vi "ui_DataLog Query Large String.vi"(0 "prompt":string, 7 "string in (\"\")":string) -> (4 "OKed?":bool, 8 "string out":string)   [LabVIEW 2012]
doc: "This dialog queries for a large string. The titlebar indicates what kind of string is expected."
uses:
  typedefs/t_DataLog Query Large String States.ctl
panel:
  in  "string":string
  in  "cancel":bool
  in  "OK":bool
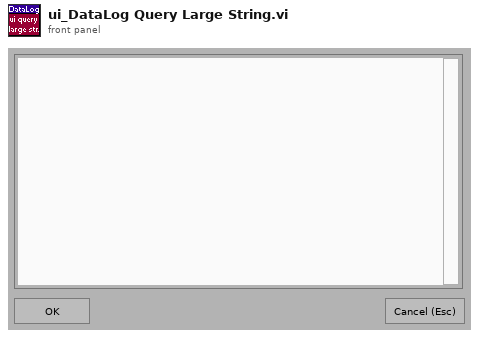
[diagram p1: front panel]
types:
  T1 = typedef "t_DataLog Query Large String States.ctl" = enum16{"empty queue", "initialize", "stop"}
  T2 = typedef "eventvkey.ctl" = enum16{"ASCII", "Enter", "Return", "Shift", "Ctrl", "Alt", "Cmd", "Opt", "Caps", "NumLock", "Clear", "Break", "Up", "Down", "Left", "Right", "Insert", "Delete", "Home", "End", "PageUp", "PageDown", "Escape", "Help", "Pause", "ScrollLock", "F1", "F2", "F3", "F4", "F5", "F6", "F7", "F8", "F9", "F10", "F11", "F12", "F13", "F14", "F15", "F16", "F17", "F18", "F19", "F20", "F21", "F22", "F23", "F24", "Play", "VolumeUp", "VolumeDown", "Mute", "Two Byte Char"}
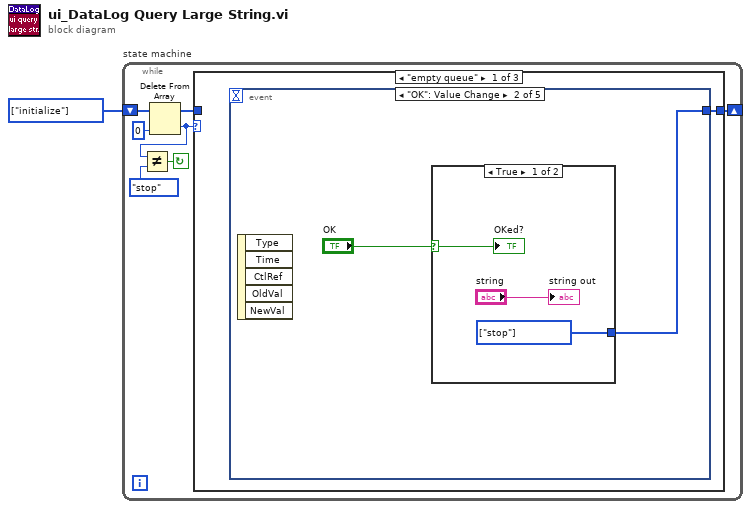
[diagram p0: block diagram]
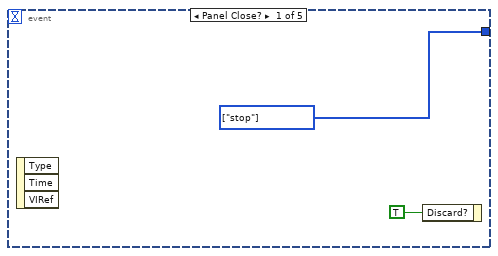
[diagram p2: hidden frame]
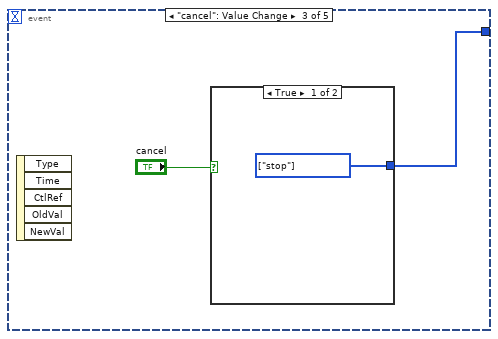
[diagram p4: hidden frame]
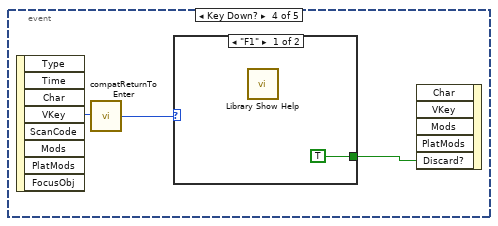
[diagram p6: hidden frame]
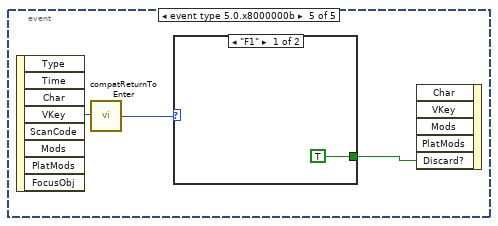
[diagram p8: hidden frame]
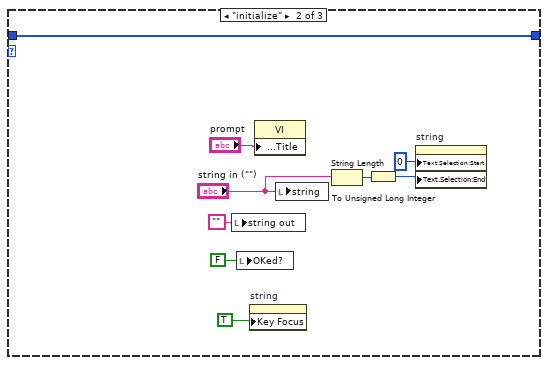
[diagram p10: hidden frame]
diagram:
  w1 = T1[] [enum."initialize"] items=["empty queue", "initialize", "stop"] ("Array Constant")
  n1 = while "state machine" {
    shift-left: w1 -> [w5]
    shift-right: [w8] -> _
    stop <- w7 continue-if-true
    n2 = Delete From Array(array=w5, index=0) -> (deleted portion=w3:T1, array with subset deleted=w4:T1[])  [unwired: 1 in]
    n3 = Not Equal?(x=w3, y=t_DataLog_Query_Large_String_States."stop" ("states")) -> (x != y?=w7:bool)
    n4 = case "Case" shown="\"empty queue\"" w3 {
      tunnel: [w9 w36 w37] -> w8
      tunnel: w4 -> [_ w36 w37]
      frame "empty queue" {
        n5 = event shown="[1] \"OK\": Value Change" {
          selector: _ -> [_ _ _ _ _]
          dyn-events: _ -> [_ _ _ _ _]
          timeout: _ -> [_ _ _ _ _]
          tunnel: [w11 w13 w18 _ _] -> w9
          event Panel Close? {
            w11 = T1[] [enum."stop"] items=["empty queue", "initialize", "stop"] ("Array Constant")
            n6 = event-data() -> ()  [unwired: 1 in, 3 out]
            n7 = event-data("Discard?"=TRUE) -> ()  [unwired: 1 in, 1 out]
          }
          event "OK": Value Change {
            n8 = event-data() -> ()  [unwired: 1 in, 5 out]
            n9 = case shown="True" "OK" {
              selector: "OK" -> [w14 _]
              tunnel: [w16 _] -> w13
              frame True {
                w16 = T1[] [enum."stop"] items=["empty queue", "initialize", "stop"] ("Array Constant")
                "string out" <- "string"
                "OKed?" <- w14
              }
              frame False {
              }
            }
          }
          event "cancel": Value Change {
            n10 = event-data() -> ()  [unwired: 1 in, 5 out]
            n11 = case shown="True" "cancel" {
              tunnel: [w19 _] -> w18
              frame True {
                w19 = T1[] [enum."stop"] items=["empty queue", "initialize", "stop"] ("Array Constant")
              }
              frame False {
              }
            }
          }
          event Key Down? {
            n12 = event-data() -> ("VKey"=w20:T2)  [unwired: 1 in, 7 out]
            n13 = call <vilib>:"compatReturnToEnter.vi"("VKey"=w20) -> ("VKey"=w22:T2)
            n14 = case shown="\"F1\"" w22 {
              tunnel: [TRUE ("Discard?") _] -> w21
              frame "F1" {
                n15 = call "Library Show Help.vi"() -> ()  [unwired: 1 in]
              }
              frame Default {
              }
            }
            n16 = event-data("Discard?"=w21) -> ()  [unwired: 5 in, 1 out]
          }
          event event type 5.0.x8000000b {
            n17 = event-data() -> ("VKey"=w24:T2)  [unwired: 1 in, 7 out]
            n18 = call <vilib>:"compatReturnToEnter.vi"("VKey"=w24) -> ("VKey"=w26:T2)
            n19 = case shown="\"F1\"" w26 {
              tunnel: [TRUE ("Discard?") _] -> w25
              frame "F1" {
              }
              frame Default {
              }
            }
            n20 = event-data("Discard?"=w25) -> ()  [unwired: 5 in, 1 out]
          }
        }
      }
      frame "initialize" {
        n21 = local write "string out"("" ("result")) -> ()
        n22 = local write "OKed?"(FALSE ("OKed?")) -> ()
        n23 = property on="string" class="Str"("Key Focus"=TRUE) -> ()  [unwired: 2 in, 2 out]
        n24 = property class="VI"("Front Panel Window:Title"="prompt") -> ()  [unwired: 2 in, 2 out]
        n25 = local write "string"("string in (\"\")") -> ()
        n26 = String Length(string="string in (\"\")") -> (length=w31:i32)
        n27 = To Unsigned Long Integer(number=w31) -> (unsigned 32bit integer=w28:u32)
        n28 = property on="string" class="Str"("Text.Selection:Start"=u32 0, "Text.Selection:End"=w28) -> ()  [unwired: 2 in, 2 out]
      }
      frame "stop" {
      }
    }
  }
